vi "Merge Status.vi"(10 "New":T1, 11 "Current":T1) -> (3 "Status":T1=enum."Passed")   [LabVIEW 2020, in "Execution API.lvclass"]
uses:
  Execution API.lvclass
  Core/Result/Status.ctl
  Core/Result/Result.lvlib
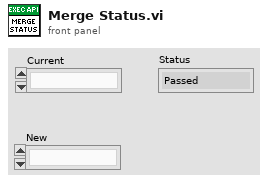
[diagram p1: front panel]
types:
  T1 = typedef "Result.lvlib/Status.ctl" = enum16{"", "Passed", "Failed", "Error", "Skipped", "Setup Error", "Broken", "Teardown Error"}
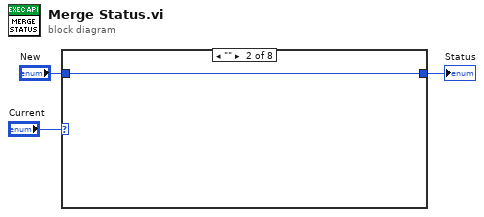
[diagram p0: block diagram]
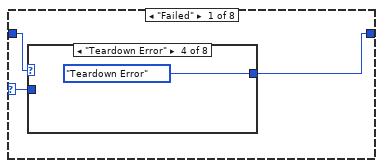
[diagram p2: hidden frame]
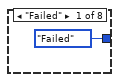
[diagram p3: hidden frame]
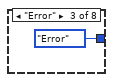
[diagram p5: hidden frame]
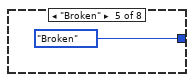
[diagram p6: hidden frame]
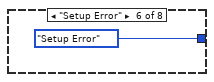
[diagram p7: hidden frame]
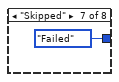
[diagram p8: hidden frame]
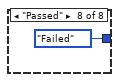
[diagram p9: hidden frame]
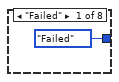
[diagram p11: hidden frame]
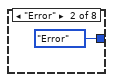
[diagram p12: hidden frame]
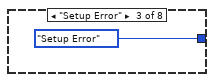
[diagram p13: hidden frame]
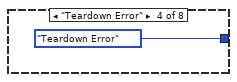
[diagram p14: hidden frame]
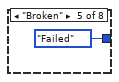
[diagram p15: hidden frame]
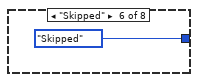
[diagram p16: hidden frame]
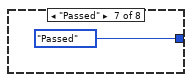
[diagram p17: hidden frame]
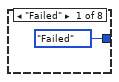
[diagram p19: hidden frame]
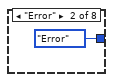
[diagram p20: hidden frame]
diagram:
  n1 = case shown="\"\"" "Current" {
    selector: "Current" -> [w4 _ w16 w27 _ _ _ _]
    tunnel: "New" -> [w6 w15 w18 w29 _ _ w40 w44]
    tunnel: [w5 w15 w17 w28 Status."Error" ("Merged Status") Status."Setup Error" ("Merged Status") w41 w44] -> w3
    frame "Failed" {
      n2 = case shown="\"Teardown Error\"" w6 {
        tunnel: [Status."Failed" ("Merged Status") w8 Status."Error" ("Merged Status") Status."Teardown Error" ("Merged Status") Status."Broken" ("Merged Status") Status."Setup Error" ("Merged Status") Status."Failed" ("Merged Status") Status."Failed" ("Merged Status")] -> w5
        tunnel: w4 -> [_ w8 _ _ _ _ _ _]
        frame "Failed" {
        }
        frame "" {
        }
        frame "Error" {
        }
        frame "Teardown Error" {
        }
        frame "Broken" {
        }
        frame "Setup Error" {
        }
        frame "Skipped" {
        }
        frame "Passed" {
        }
      }
    }
    frame "" {
    }
    frame "Skipped" {
      n3 = case shown="\"\"" w18 {
        tunnel: [Status."Failed" ("Merged Status") Status."Error" ("Merged Status") Status."Setup Error" ("Merged Status") Status."Teardown Error" ("Merged Status") Status."Failed" ("Merged Status") Status."Skipped" ("Merged Status") Status."Passed" ("Merged Status") w26] -> w17
        tunnel: w16 -> [_ _ _ _ _ _ _ w26]
        frame "Failed" {
        }
        frame "Error" {
        }
        frame "Setup Error" {
        }
        frame "Teardown Error" {
        }
        frame "Broken" {
        }
        frame "Skipped" {
        }
        frame "Passed" {
        }
        frame "" {
        }
      }
    }
    frame "Passed" {
      n4 = case shown="\"\"" w29 {
        tunnel: [Status."Failed" ("Merged Status") Status."Error" ("Merged Status") Status."Setup Error" ("Merged Status") Status."Failed" ("Merged Status") Status."Teardown Error" ("Merged Status") Status."Passed" ("Merged Status") w36 Status."Passed" ("Merged Status")] -> w28
        tunnel: w27 -> [_ _ _ _ _ _ w36 _]
        frame "Failed" {
        }
        frame "Error" {
        }
        frame "Setup Error" {
        }
        frame "Broken" {
        }
        frame "Teardown Error" {
        }
        frame "Skipped" {
        }
        frame "" {
        }
        frame "Passed" {
        }
      }
    }
    frame "Error" {
    }
    frame "Setup Error" {
    }
    frame "Teardown Error" {
      n5 = case shown="\"Error\", \"Setup Error\", \"Broken\"" w40 {
        selector: w40 -> [_ w43]
        tunnel: [Status."Teardown Error" ("Merged Status") w43] -> w41
        frame Default {
        }
        frame "Error", "Setup Error", "Broken" {
        }
      }
    }
    frame "Broken" {
    }
  }
  "Status" <- w3
